vi "ShoulderRestPosConstant.vi"() -> (3 "RestPosition":dbl)   [LabVIEW 2023]
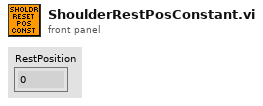
[diagram p1: front panel]
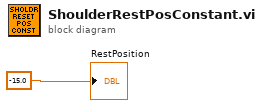
[diagram p0: block diagram]
diagram:
  "RestPosition" <- -15.0 ("Position")
